vi "Read Decrement Key Binding.vi"(9 "Numeric in":refnum<class "Numeric.lvclass">) -> (3 "Numeric out":refnum<class "Numeric.lvclass">, 4 "Decrement Key Binding":T1)   [LabVIEW 2014, in "Raspberry Pi Compatible Compiler for LabVIEW.lvlib" / "Numeric.lvclass"]
uses:
  Numeric.lvclass
  <vilib>/Utility/miscctls.llb/LVKeyTypeDef.ctl
  Numeric.lvclass/Numeric.ctl
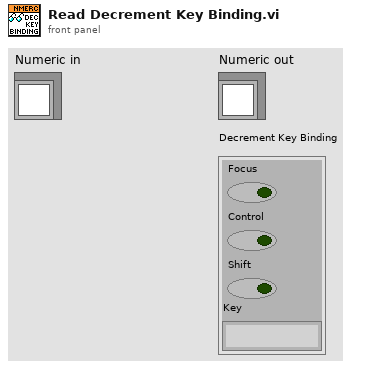
[diagram p1: front panel]
types:
  T1 = typedef "LVKeyTypeDef.ctl" = cluster{"Focus":bool, "Control":bool, "Shift":bool, "Key":string}
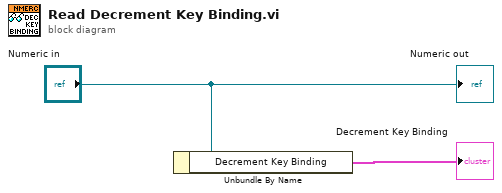
[diagram p0: block diagram]
diagram:
  n1 = Unbundle By Name("Numeric in") -> ("Decrement Key Binding"=→"Decrement Key Binding":T1)
  "Numeric out" <- "Numeric in"
